vi "Client Create.vi"(8 "error in (no error)":errorcluster, 11 "Telegram Class in":refnum<class "Telegram Class.lvclass">) -> (0 "error out":errorcluster, 3 "Telegram Class out":refnum<class "Telegram Class.lvclass">)   [LabVIEW 2015, in "Telegram Library.lvlib" / "Telegram Class.lvclass"]
doc: "Created IvanLis by LabVIEW Portal\nProfile: http://labviewportal.org/memberlist.php?mode=viewprofile&u=987\neMail: IvanLisanov@gMail.com\nTelegram: https://t.me/IvanLis"
uses:
  Telegram Class.lvclass
  Telegram Class.lvclass/Telegram Class.ctl
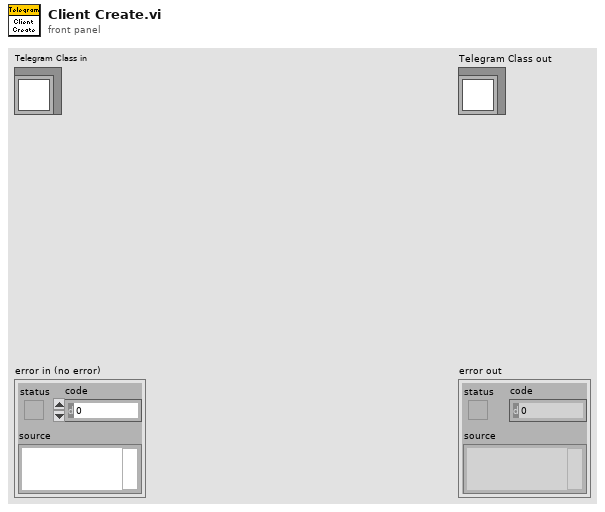
[diagram p1: front panel]
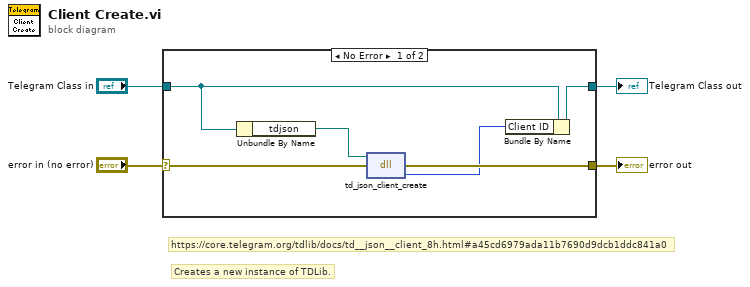
[diagram p0: block diagram]
diagram:
  # "Creates a new instance of TDLib."
  # "https://core.telegram.org/tdlib/docs/td__json__client_8h.html#a45cd6979ada11b7690d9dcb1ddc841a0"
  n1 = case shown="No Error" "error in (no error)" {
    selector: "error in (no error)" -> [w10 w12]
    tunnel: [w9 w12] -> w3
    tunnel: [w6 w11] -> w1
    tunnel: "Telegram Class in" -> [w8 w11]
    frame No Error {
      n2 = Unbundle By Name(w8) -> ("tdjson"=w7:path)
      n3 = dll-call lib="C:/Users/Ivan/Desktop/Telegram/Project/DLL/tdjson-x32.dll" fn="td_json_client_create"(path in=w7, error in=w10) -> (error out=w9:errorcluster, "Client ID"=w5:i32)  [unwired: 1 in, 1 out]
      n4 = Bundle By Name(cluster=w8, "Client ID"=w5) -> (w6:refnum<class "Telegram Class.lvclass">)
    }
    frame Error {
    }
  }
  "error out" <- w3
  "Telegram Class out" <- w1
